vi "updateTrialInfo (SubVI).vi"(4 "data Path":path, 5 "Protocol":T1, 7 "currentBlockInfo":T7={"BlockInfo"={"block #"=0, "block cond"=enum."RHP", "Trial # in block"=0}, "Trial #"=0}) -> (0 "file path out":path, 1 "dCOP cond":T5 items=["all off"=0, "all on"=63, "0 mm"=1, "+8.84 mm"=2, "+15.76 mm"=3, "+22.68 mm"=4, "+29.60 mm"=5, "+36.52 mm"=6, "+43.44 mm"=7, "+50.36 mm"=8, "+57.28 mm"=9, "+64.20 mm"=10, "-8.84 mm"=11, "-15.76 mm"=12, "-22.68 mm"=13, "-29.60 mm"=14, "-36.52 mm"=15, "-43.44 mm"=16, "-50.36 mm"=17, "-57.28 mm"=18, "-64.20 mm"=19], 2 "CM cond":T6, 3 "next":T7={"BlockInfo"={"block #"=0, "block cond"=enum."RHP", "Trial # in block"=0}, "Trial #"=0})   [LabVIEW 2021]
uses:
  ctrTrialInfo.ctl
  ctrBlockInfo.ctl
  ctrBlockCondition.ctl
  ctrCMCondition.ctl
  ctrLED_R2L.ctl
  ctlProtocol.ctl
  ctlProtocolSubID.ctl
  ctlBlockOrder.ctl
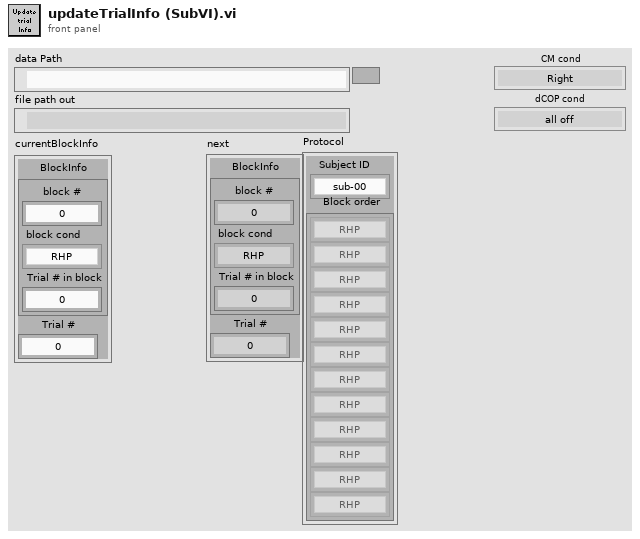
[diagram p1: front panel]
types:
  T1 = typedef "ctlProtocol.ctl" = cluster{"Subject ID":T2, "Block order":T3}
  T2 = typedef "ctlProtocolSubID.ctl" = enum16{"sub-00", "sub-01", "sub-02", "sub-03", "sub-04", "sub-05", "sub-06", "sub-07", "sub-08", "sub-09", "sub-10", "sub-11", "sub-12", "sub-13", "sub-14", "sub-15", "sub-16", "sub-17", "sub-18", "sub-19", "sub-20", "sub-21", "sub-22", "sub-23", "sub-24", "sub-25", "sub-26", "sub-27", "sub-28", "sub-29", "sub-30", "sub-31", "sub-32", "sub-33", "sub-34", "sub-35", "sub-36", "sub-37", "sub-38", "sub-39", "sub-40"}
  T3 = typedef "ctlBlockOrder.ctl" = T4[]
  T4 = typedef "ctrBlockCondition.ctl" = enum16{"famDrop", "preDrop", "famTask", "RHP", "RLD", "RHD", "LHP", "LLD", "LHD", "UR", "UL", "pstDrop"}
  T5 = typedef "ctrLED_R2L.ctl" = u16
  T6 = typedef "ctrCMCondition.ctl" = enum16{"Right", "Center", "Left"}
  T7 = typedef "ctrTrialInfo.ctl" = cluster{"BlockInfo":T8, "Trial #":i32}
  T8 = typedef "ctrBlockInfo.ctl" = cluster{"block #":i32, "block cond":T4, "Trial # in block":i32}
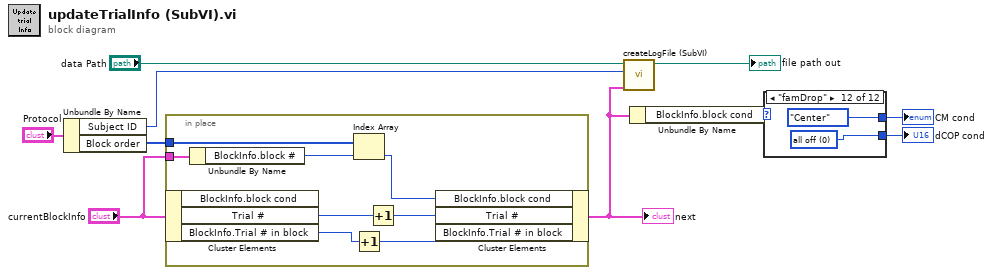
[diagram p0: block diagram]
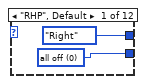
[diagram p2: hidden frame]
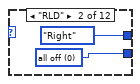
[diagram p3: hidden frame]
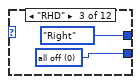
[diagram p4: hidden frame]
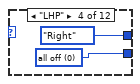
[diagram p5: hidden frame]
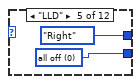
[diagram p6: hidden frame]
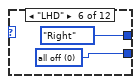
[diagram p7: hidden frame]
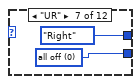
[diagram p8: hidden frame]
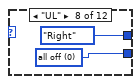
[diagram p9: hidden frame]
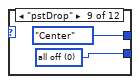
[diagram p10: hidden frame]
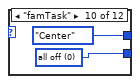
[diagram p11: hidden frame]
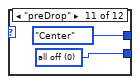
[diagram p12: hidden frame]
diagram:
  n1 = Unbundle By Name("Protocol") -> ("Subject ID"=w5:T2, "Block order"=w3:T3)
  n2 = in-place {
    in-place-border: "currentBlockInfo" -> [w15]
    in-place-border: w3 -> [w14]
    n3 = in-place-cluster #1("currentBlockInfo") -> ("Trial #"=w17:i32, "BlockInfo.Trial # in block"=w18:i32)  [unwired: 1 out]
    n4 = Unbundle By Name(w15) -> ("BlockInfo.block #"=w13:i32)
    n5 = Index Array(array=w14, index=w13) -> (element=w12:T4)
    n6 = Increment(x=w18) -> (x+1=w11:i32)
    n7 = Increment(x=w17) -> (x+1=w16:i32)
    n8 = in-place-cluster #1("BlockInfo.block cond"=w12, "Trial #"=w16, "BlockInfo.Trial # in block"=w11) -> (w2:T7)
  }
  "next" <- w2
  n9 = call "createLogFile (SubVI).vi"("TrialInfo"=w2, "Subject ID"=w5, "directory Path"="data Path") -> ("file path out"=→"file path out":path)  [unwired: 8 in]
  n10 = Unbundle By Name(w2) -> ("BlockInfo.block cond"=w1:T4)
  n11 = case shown="\"famDrop\"" w1 {
    tunnel: [w19 w21 w23 w25 w27 w29 w31 w33 w35 w37 w39 w41] -> w8
    tunnel: [ctrCMCondition."Right" ("CM cond") ctrCMCondition."Right" ("CM cond") ctrCMCondition."Right" ("CM cond") ctrCMCondition."Right" ("CM cond") ctrCMCondition."Right" ("CM cond") ctrCMCondition."Right" ("CM cond") ctrCMCondition."Right" ("CM cond") ctrCMCondition."Right" ("CM cond") ctrCMCondition."Center" ("CM cond") ctrCMCondition."Center" ("CM cond") ctrCMCondition."Center" ("CM cond") ctrCMCondition."Center" ("CM cond")] -> w9
    frame "RHP", Default {
      w19 = T5 0 items=["all off"=0, "all on"=63, "0 mm"=1, "+8.84 mm"=2, "+15.76 mm"=3, "+22.68 mm"=4, "+29.60 mm"=5, "+36.52 mm"=6, "+43.44 mm"=7, "+50.36 mm"=8, "+57.28 mm"=9, "+64.20 mm"=10, "-8.84 mm"=11, "-15.76 mm"=12, "-22.68 mm"=13, "-29.60 mm"=14, "-36.52 mm"=15, "-43.44 mm"=16, "-50.36 mm"=17, "-57.28 mm"=18, "-64.20 mm"=19, "CM Right"=20, "CM Left"=21] ("dCOP cond 2")
    }
    frame "RLD" {
      w21 = T5 0 items=["all off"=0, "all on"=63, "0 mm"=1, "+8.84 mm"=2, "+15.76 mm"=3, "+22.68 mm"=4, "+29.60 mm"=5, "+36.52 mm"=6, "+43.44 mm"=7, "+50.36 mm"=8, "+57.28 mm"=9, "+64.20 mm"=10, "-8.84 mm"=11, "-15.76 mm"=12, "-22.68 mm"=13, "-29.60 mm"=14, "-36.52 mm"=15, "-43.44 mm"=16, "-50.36 mm"=17, "-57.28 mm"=18, "-64.20 mm"=19, "CM Right"=20, "CM Left"=21] ("dCOP cond 2")
    }
    frame "RHD" {
      w23 = T5 0 items=["all off"=0, "all on"=63, "0 mm"=1, "+8.84 mm"=2, "+15.76 mm"=3, "+22.68 mm"=4, "+29.60 mm"=5, "+36.52 mm"=6, "+43.44 mm"=7, "+50.36 mm"=8, "+57.28 mm"=9, "+64.20 mm"=10, "-8.84 mm"=11, "-15.76 mm"=12, "-22.68 mm"=13, "-29.60 mm"=14, "-36.52 mm"=15, "-43.44 mm"=16, "-50.36 mm"=17, "-57.28 mm"=18, "-64.20 mm"=19, "CM Right"=20, "CM Left"=21] ("dCOP cond 2")
    }
    frame "LHP" {
      w25 = T5 0 items=["all off"=0, "all on"=63, "0 mm"=1, "+8.84 mm"=2, "+15.76 mm"=3, "+22.68 mm"=4, "+29.60 mm"=5, "+36.52 mm"=6, "+43.44 mm"=7, "+50.36 mm"=8, "+57.28 mm"=9, "+64.20 mm"=10, "-8.84 mm"=11, "-15.76 mm"=12, "-22.68 mm"=13, "-29.60 mm"=14, "-36.52 mm"=15, "-43.44 mm"=16, "-50.36 mm"=17, "-57.28 mm"=18, "-64.20 mm"=19, "CM Right"=20, "CM Left"=21] ("dCOP cond 2")
    }
    frame "LLD" {
      w27 = T5 0 items=["all off"=0, "all on"=63, "0 mm"=1, "+8.84 mm"=2, "+15.76 mm"=3, "+22.68 mm"=4, "+29.60 mm"=5, "+36.52 mm"=6, "+43.44 mm"=7, "+50.36 mm"=8, "+57.28 mm"=9, "+64.20 mm"=10, "-8.84 mm"=11, "-15.76 mm"=12, "-22.68 mm"=13, "-29.60 mm"=14, "-36.52 mm"=15, "-43.44 mm"=16, "-50.36 mm"=17, "-57.28 mm"=18, "-64.20 mm"=19, "CM Right"=20, "CM Left"=21] ("dCOP cond 2")
    }
    frame "LHD" {
      w29 = T5 0 items=["all off"=0, "all on"=63, "0 mm"=1, "+8.84 mm"=2, "+15.76 mm"=3, "+22.68 mm"=4, "+29.60 mm"=5, "+36.52 mm"=6, "+43.44 mm"=7, "+50.36 mm"=8, "+57.28 mm"=9, "+64.20 mm"=10, "-8.84 mm"=11, "-15.76 mm"=12, "-22.68 mm"=13, "-29.60 mm"=14, "-36.52 mm"=15, "-43.44 mm"=16, "-50.36 mm"=17, "-57.28 mm"=18, "-64.20 mm"=19, "CM Right"=20, "CM Left"=21] ("dCOP cond 2")
    }
    frame "UR" {
      w31 = T5 0 items=["all off"=0, "all on"=63, "0 mm"=1, "+8.84 mm"=2, "+15.76 mm"=3, "+22.68 mm"=4, "+29.60 mm"=5, "+36.52 mm"=6, "+43.44 mm"=7, "+50.36 mm"=8, "+57.28 mm"=9, "+64.20 mm"=10, "-8.84 mm"=11, "-15.76 mm"=12, "-22.68 mm"=13, "-29.60 mm"=14, "-36.52 mm"=15, "-43.44 mm"=16, "-50.36 mm"=17, "-57.28 mm"=18, "-64.20 mm"=19, "CM Right"=20, "CM Left"=21] ("dCOP cond 2")
    }
    frame "UL" {
      w33 = T5 0 items=["all off"=0, "all on"=63, "0 mm"=1, "+8.84 mm"=2, "+15.76 mm"=3, "+22.68 mm"=4, "+29.60 mm"=5, "+36.52 mm"=6, "+43.44 mm"=7, "+50.36 mm"=8, "+57.28 mm"=9, "+64.20 mm"=10, "-8.84 mm"=11, "-15.76 mm"=12, "-22.68 mm"=13, "-29.60 mm"=14, "-36.52 mm"=15, "-43.44 mm"=16, "-50.36 mm"=17, "-57.28 mm"=18, "-64.20 mm"=19, "CM Right"=20, "CM Left"=21] ("dCOP cond 2")
    }
    frame "pstDrop" {
      w35 = T5 0 items=["all off"=0, "all on"=63, "0 mm"=1, "+8.84 mm"=2, "+15.76 mm"=3, "+22.68 mm"=4, "+29.60 mm"=5, "+36.52 mm"=6, "+43.44 mm"=7, "+50.36 mm"=8, "+57.28 mm"=9, "+64.20 mm"=10, "-8.84 mm"=11, "-15.76 mm"=12, "-22.68 mm"=13, "-29.60 mm"=14, "-36.52 mm"=15, "-43.44 mm"=16, "-50.36 mm"=17, "-57.28 mm"=18, "-64.20 mm"=19, "CM Right"=20, "CM Left"=21] ("dCOP cond 2")
    }
    frame "famTask" {
      w37 = T5 0 items=["all off"=0, "all on"=63, "0 mm"=1, "+8.84 mm"=2, "+15.76 mm"=3, "+22.68 mm"=4, "+29.60 mm"=5, "+36.52 mm"=6, "+43.44 mm"=7, "+50.36 mm"=8, "+57.28 mm"=9, "+64.20 mm"=10, "-8.84 mm"=11, "-15.76 mm"=12, "-22.68 mm"=13, "-29.60 mm"=14, "-36.52 mm"=15, "-43.44 mm"=16, "-50.36 mm"=17, "-57.28 mm"=18, "-64.20 mm"=19, "CM Right"=20, "CM Left"=21] ("dCOP cond 2")
    }
    frame "preDrop" {
      w39 = T5 0 items=["all off"=0, "all on"=63, "0 mm"=1, "+8.84 mm"=2, "+15.76 mm"=3, "+22.68 mm"=4, "+29.60 mm"=5, "+36.52 mm"=6, "+43.44 mm"=7, "+50.36 mm"=8, "+57.28 mm"=9, "+64.20 mm"=10, "-8.84 mm"=11, "-15.76 mm"=12, "-22.68 mm"=13, "-29.60 mm"=14, "-36.52 mm"=15, "-43.44 mm"=16, "-50.36 mm"=17, "-57.28 mm"=18, "-64.20 mm"=19, "CM Right"=20, "CM Left"=21] ("dCOP cond 2")
    }
    frame "famDrop" {
      w41 = T5 0 items=["all off"=0, "all on"=63, "0 mm"=1, "+8.84 mm"=2, "+15.76 mm"=3, "+22.68 mm"=4, "+29.60 mm"=5, "+36.52 mm"=6, "+43.44 mm"=7, "+50.36 mm"=8, "+57.28 mm"=9, "+64.20 mm"=10, "-8.84 mm"=11, "-15.76 mm"=12, "-22.68 mm"=13, "-29.60 mm"=14, "-36.52 mm"=15, "-43.44 mm"=16, "-50.36 mm"=17, "-57.28 mm"=18, "-64.20 mm"=19, "CM Right"=20, "CM Left"=21] ("dCOP cond 2")
    }
  }
  "CM cond" <- w9
  "dCOP cond" <- w8
